vi "Resize Window.vi"(8 "Error in":errorcluster, 10 "Front Panel Window:Panel Bounds":T1, 11 "VI reference in":refnum<vi>) -> (0 "Error out":errorcluster, 3 "VI reference out":refnum<vi>)   [LabVIEW 2019]
uses:
  <vilib>/Utility/miscctls.llb/LVRectTypeDef.ctl
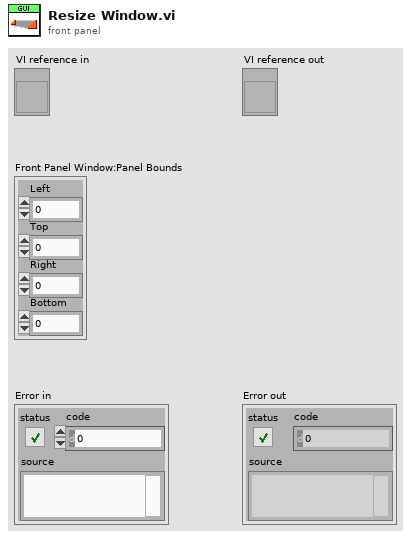
[diagram p1: front panel]
types:
  T1 = typedef "LVRectTypeDef.ctl" = cluster{"Left":i16, "Top":i16, "Right":i16, "Bottom":i16}
  T2 = enum32{"Invalid", "Standard", "Closed", "Hidden", "Minimized", "Maximized"}
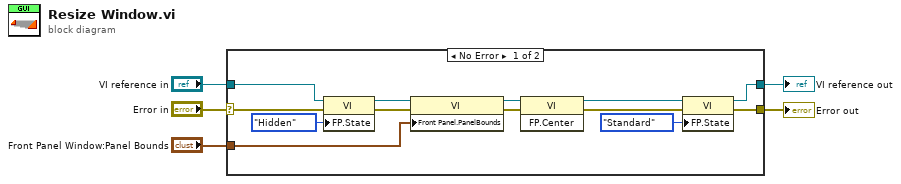
[diagram p0: block diagram]
diagram:
  n1 = case shown="No Error" "Error in" {
    selector: "Error in" -> [w16 w19]
    tunnel: "VI reference in" -> [w9 w20]
    tunnel: [w13 w20] -> w3
    tunnel: [w12 w19] -> w2
    tunnel: "Front Panel Window:Panel Bounds" -> [w6 _]
    frame No Error {
      n2 = property class="VI"(reference=w9, error in=w16, "FP.State"=T2."Hidden" ("Front Panel Window:State")) -> (reference out=w8:refnum<vi>, error out=w7:errorcluster)
      n3 = property class="VI"(reference=w8, error in=w7, "Front Panel.PanelBounds"=w6) -> (reference out=w15:refnum<vi>, error out=w10:errorcluster)
      n4 = invoke class="VI" method="FP.Center"(reference=w15, error in=w10) -> (reference out=w14:refnum<vi>, error out=w11:errorcluster)  [unwired: 1 in, 1 out]
      n5 = property class="VI"(reference=w14, error in=w11, "FP.State"=T2."Standard" ("Front Panel Window:State")) -> (reference out=w13:refnum<vi>, error out=w12:errorcluster)
    }
    frame Error {
    }
  }
  "Error out" <- w2
  "VI reference out" <- w3
